vi "Create_NNFE_Paths_From_Folder.vi"(11 "NNFE_Folder_Paths":path[](array[path])) -> (3 "NNFE_File_Paths":T1[](array[typedef]))   [LabVIEW 2020]
uses:
  <vilib>/Ngene/DeepLTK Anomaly Detection Addon/DeepLTK_Anomaly_Detection_Addon/API/Controls/NN_Paths.ctl
  <vilib>/Ngene/DeepLTK Anomaly Detection Addon/DeepLTK_Anomaly_Detection_Addon/DeepLTK_Anomaly_Detection_Addon.lvlib
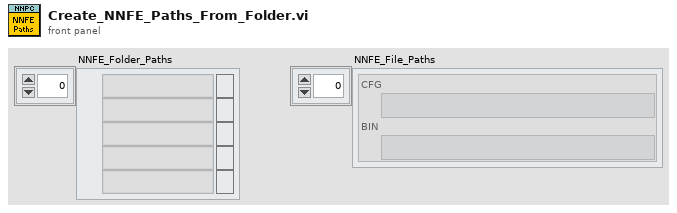
[diagram p1: front panel]
types:
  T1 = typedef "DeepLTK_Anomaly_Detection_Addon.lvlib/NN_Paths.ctl" = cluster{"CFG":path, "BIN":path}
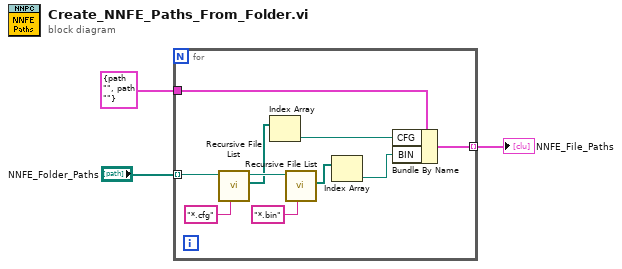
[diagram p0: block diagram]
diagram:
  n1 = for {
    tunnel: "NNFE_Folder_Paths" -> [w13] mode=indexing
    tunnel: T1 {"CFG"=path "", "BIN"=path ""} ("NNFE_Paths") -> [w9]
    tunnel: [w4] -> w2 mode=indexing
    n2 = call <vilib>:"Recursive File List.vi"("pattern"="*.cfg", "Folder Path"=w13) -> ("All Files in Dir"=w5:path[], "dup Folder Path"=w10:path)  [unwired: 5 in, 3 out]
    n3 = Index Array(array=w5) -> (element=w6:path)  [unwired: 1 in]
    n4 = call <vilib>:"Recursive File List.vi"("pattern"="*.bin", "Folder Path"=w10) -> ("All Files in Dir"=w7:path[])  [unwired: 5 in, 4 out]
    n5 = Index Array(array=w7) -> (element=w8:path)  [unwired: 1 in]
    n6 = Bundle By Name(cluster=w9, "CFG"=w6, "BIN"=w8) -> (w4:T1)
  }
  "NNFE_File_Paths" <- w2
